vi "Draw.vi"(0 "reference in":refnum<class "Map.lvclass">, 1 "PictureIn":picture, 5 "error in (no error)":errorcluster) -> (14 "reference out":refnum<class "Map.lvclass">, 15 "PictureOut":picture, 19 "error out":errorcluster)   [LabVIEW 2016, in "Map.lvclass"]
doc: "Draws the MAP"
uses:
  Map.lvclass
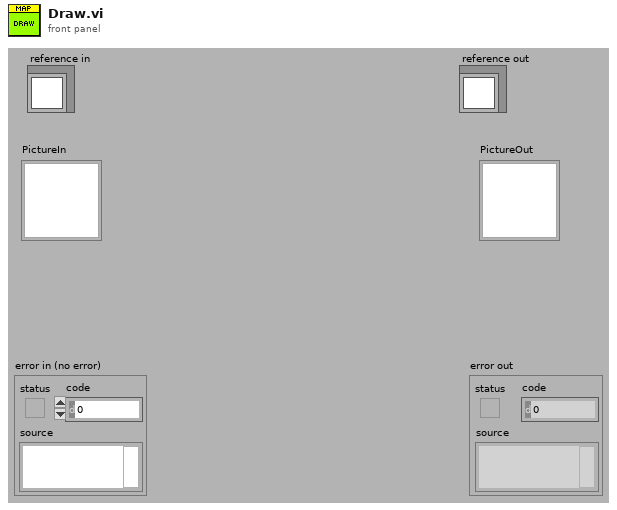
[diagram p1: front panel]
types:
  T1 = typedef "Map.lvclass/ObjectAttributes.ctl" = cluster{"Width":i32, "Height":i32, "Map":bool[][]}
  T2 = typedef "imagedata.ctl" = cluster{"image type":i32, "image depth":i32, "image":u8[], "mask":u8[], "colors":u32[], "Rectangle":cluster{"left":i16, "top":i16, "right":i16, "bottom":i16}}
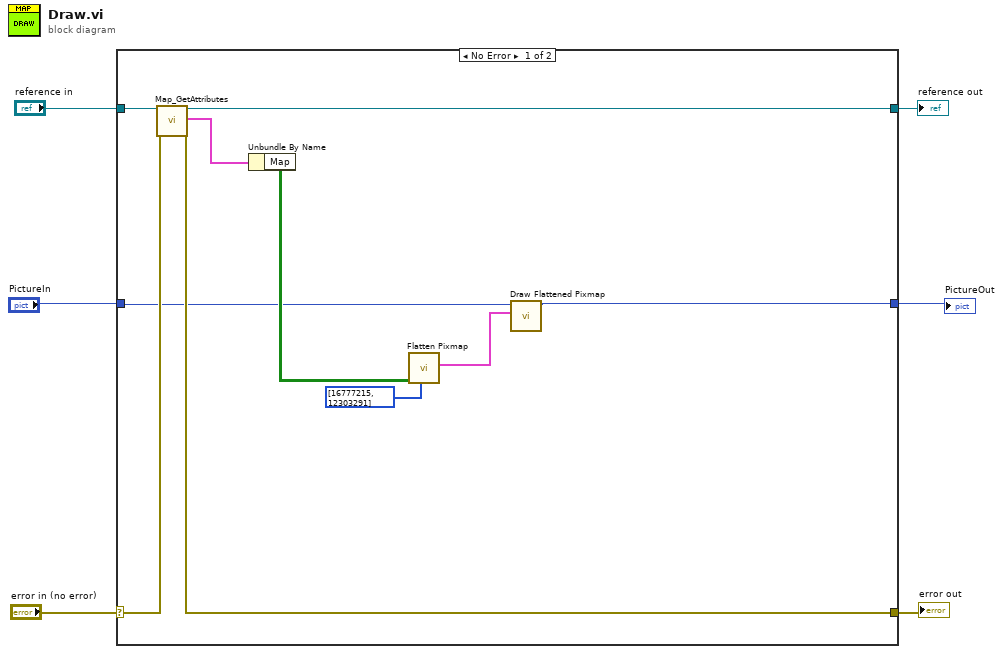
[diagram p0: block diagram]
diagram:
  n1 = case shown="No Error" "error in (no error)" {
    selector: "error in (no error)" -> [w16 w19]
    tunnel: [w15 w19] -> w5
    tunnel: [w13 w18] -> w3
    tunnel: "reference in" -> [w14 w18]
    tunnel: "PictureIn" -> [w9 w17]
    tunnel: [w8 w17] -> w1
    frame No Error {
      n2 = call "Map_GetAttributes.vi"("reference in"=w14, "error in (no error)"=w16) -> ("reference out"=w13:refnum<class "Map.lvclass">, "Attributes"=w11:T1, "error out"=w15:errorcluster)  [unwired: 15 out]
      n3 = Unbundle By Name(w11) -> ("Map"=w10:bool[][])
      n4 = call <vilib>:"Flatten Pixmap.vi"("colors"=u32[] [16777215, 12303291], "1-bit pixmap"=w10) -> ("image data"=w12:T2)  [unwired: 4 in, 5 out]
      n5 = call <vilib>:"Draw Flattened Pixmap.vi"("image data"=w12, "picture"=w9) -> ("new picture"=w8:picture)  [unwired: 7 out]
    }
    frame Error {
    }
  }
  "error out" <- w5
  "reference out" <- w3
  "PictureOut" <- w1
